vi "SendBufferIn.vi"(1 "remote":bool, 2 "ID":u32 format="%04x", 4 "ExtFrame":bool, 5 "数据":u8[](array[numeric])) -> ()   [LabVIEW 2011]
uses:
  _USB_CAN_SEND_BUFF_UNIT_.ctl
  _USB_CAN_GLOBAL_.vi
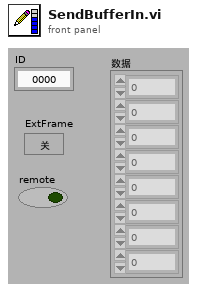
[diagram p1: front panel]
types:
  T1 = typedef "_USB_CAN_SEND_BUFF_UNIT_.ctl" = cluster{"datalen":u8, "data":u8[], "id":u8[], "extended":bool, "remote":bool}
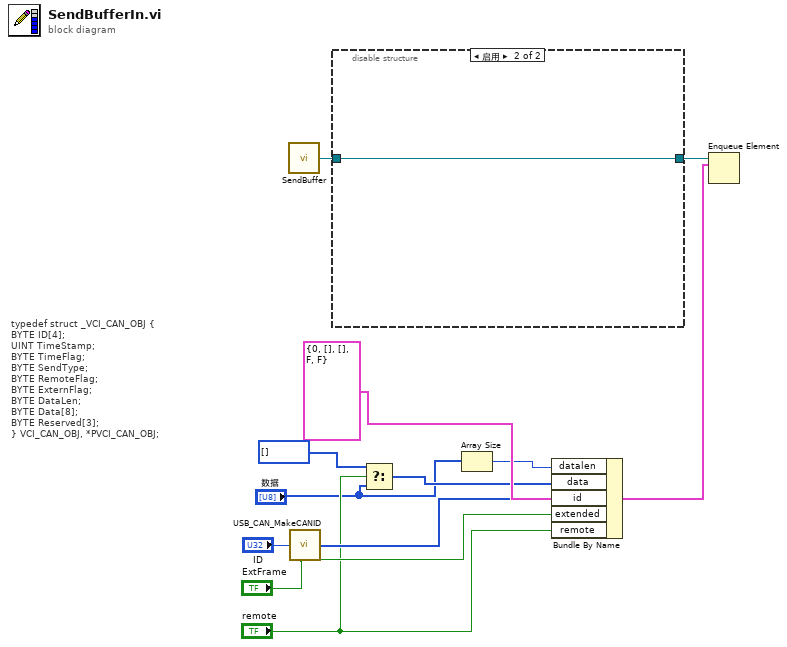
[diagram p0: block diagram]
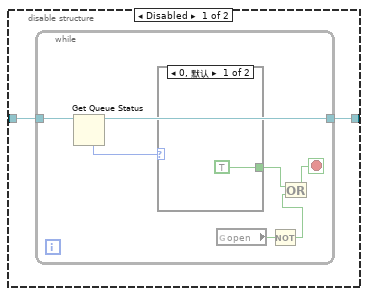
[diagram p2: hidden frame]
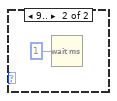
[diagram p3: hidden frame]
diagram:
  # "typedef struct _VCI_CAN_OBJ { \nBYTE ID[4];\nUINT TimeStamp; \nBYTE TimeFlag;\nBYTE SendType; \nBYTE RemoteFlag; \nBYTE ExternFlag; \nBYTE DataLen; \nBYTE Data[8]; \nBYTE Reserved[3];\n} VCI_CAN_OBJ, *PVCI_CAN_OBJ;"
  n1 = call "SendBuffer.vi"() -> ("VCI_CAN_BUF_T"=w7:refnum<queue>)  [unwired: 1 in]
  n2 = call "USB_CAN_MakeCANID.vi"("ID"="ID", "ExtFrame"="ExtFrame") -> ("IDS"=w10:u8[])  [unwired: 3 in]
  n3 = disable-structure shown="启用" {
    disable-tunnel: w7 -> [w14 w24]
    disable-tunnel: [w13 w24] -> w6
    frame Disabled {
      n4 = while {
        tunnel: w14 -> [w21]
        tunnel: [w20] -> w13
        stop <- w17 stop-if-true
        n5 = Get Queue Status(queue=w21) -> (queue out=w20:refnum<queue>, # elements in queue=w19:i32)  [unwired: 2 in, 6 out]
        n6 = case shown="0, 默认" w19 {
          tunnel: [TRUE _] -> w18
          frame 0, Default {
          }
          frame 9.. {
            n7 = Wait (ms)(milliseconds to wait=u32 1 ("等待时间（毫秒）")) -> ()  [unwired: 1 out]
          }
        }
        n8 = global read "_USB_CAN_GLOBAL_.vi" "open"() -> (w16:bool)
        n9 = Not(x=w16) -> (.not. x?=w15:bool)
        n10 = Or(x=w18, y=w15) -> (x .or. y?=w17:bool)
      }
    }
    frame Enabled {
    }
  }
  n11 = Select(t=u8[] [], s="remote", f="数据") -> (s? t:f=w2:u8[])
  n12 = Array Size(array="数据") -> (size(s)=w8:i32)
  n13 = Bundle By Name(cluster=T1 {"datalen"=0, "data"=[], "id"=[], "extended"=FALSE, "remote"=FALSE} ("VCI_CAN_BUF_T"), "datalen"=w8, "data"=w2, "id"=w10, "extended"="ExtFrame", "remote"="remote") -> (w5:T1)
  n14 = Enqueue Element(queue=w6, element=w5) -> ()  [unwired: 2 in, 3 out]
